vi "clear Session Data.vi"(0 "FPGA In":refnum<class "Exscalabar FPGA.lvclass">, 11 "error in":errorcluster) -> (4 "FPGA Out":refnum<class "Exscalabar FPGA.lvclass">, 15 "error out":errorcluster)   [LabVIEW 2014, in "Exscalabar FPGA.lvclass"]
doc: "On exit, stop the operation of the FPGA and close the reference to the FPGA session."
uses:
  Exscalabar FPGA.lvclass
  Exscalabar FPGA.lvclass/Exscalabar FPGA.ctl
  reusable/Session APIs/Session Log/System Log.lvclass
  Read Ex FPGA Ref.vi
  Read logSession.vi
  <vilib>/FPGAPlugInAG/PXI-7842R/niLvFpga_Close_PXI-7842R.vi
  <vilib>/rvi/errors/niLvFpgaAdjustHostInterfaceError.vi
  <vilib>/Utility/error.llb/Error Cluster From Error Code.vi
  <vilib>/rvi/interface/nirviCloseFPGA/nirviCloseFPGA.xnode
  R FPGA Ref.ctl
  FPGA Bitfiles/FPGAServerV2.lvbitx
  <vilib>/rvi/interface/nirviReadWriteControl/nirviReadWriteControl.xnode
  <userlib>/_Session Fwk/Session - Root.lvclass
  PAS/ePAS Library.lvlib
  NiFpgaLv.dll
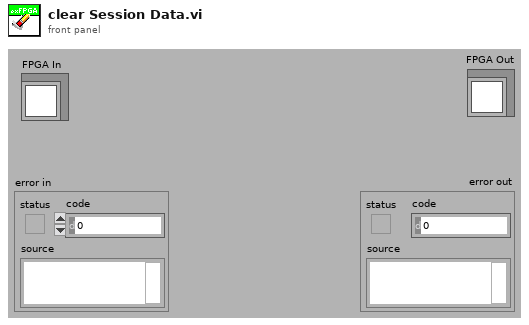
[diagram p1: front panel]
types:
  T1 = typedef "ePAS Library.lvlib/R FPGA Ref.ctl" = refnum<k20>
  T2 = typedef "Session - Root.lvclass/Session Handle.ctl" = refnum<data-value>
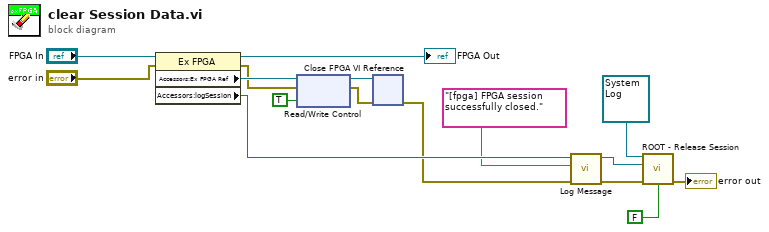
[diagram p0: block diagram]
diagram:
  n1 = property class="Ex FPGA"(reference="FPGA In", error in="error in") -> (reference out=→"FPGA Out":refnum<class "Exscalabar FPGA.lvclass">, error out=w11:errorcluster, "Accessors:Ex FPGA Ref"=w14:T1, "Accessors:logSession"=w8:T2)
  n2 = xnode "Read/Write Control"("FPGA VI Reference In"=w14, "error in"=w11, "stop"=TRUE) -> ("FPGA VI Reference Out"=w10:T1, "error out"=w9:errorcluster)
  n3 = xnode "Close FPGA VI Reference"("FPGA VI Reference In"=w10, "error in"=w9) -> ("error out"=w6:errorcluster)
  n4 = call "Log Message.vi"("error in"=w6, "MSG In"="[fpga] FPGA session successfully closed.", "session in"=w8) -> ("error out"=w5:errorcluster, "session out"=w2:T2)  [unwired: 7 in]
  n5 = call <userlib>:"ROOT - Release Session.vi"("OBJ - Session in"=refnum<class "System Log.lvclass"> refnum ("Sys Log"), "Session Handle in"=w2, "error in (no error)"=w5, "force destroy? (F)"=FALSE) -> ("error out"=→"error out":errorcluster)  [unwired: 10 in, 1 out]
